vi "SetAngleCruz.vi"(0 "Time Manager Output":dbl, 1 "ta > tf/2?":bool, 2 "Angular Velocity":dbl, 3 "Time Acceleration":dbl, 4 "Time Cruise":dbl) -> (5 "Current Angle":dbl)   [LabVIEW 2015]
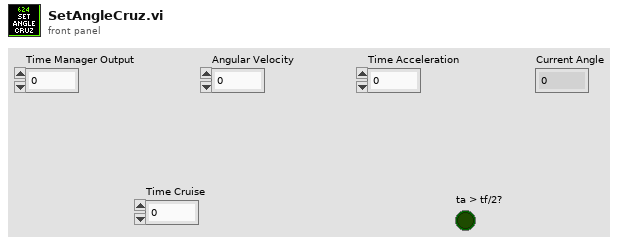
[diagram p1: front panel]
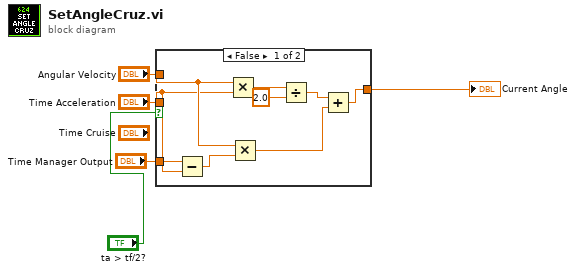
[diagram p0: block diagram]
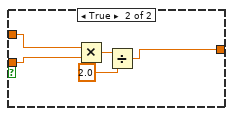
[diagram p2: hidden frame]
diagram:
  n1 = case shown="False" "ta > tf/2?" {
    tunnel: "Time Manager Output" -> [w11 _]
    tunnel: "Angular Velocity" -> [w9 w19]
    tunnel: [w7 w15] -> w3
    tunnel: "Time Acceleration" -> [w6 w18]
    frame False {
      n2 = Subtract(x=w11, y=w6) -> (x-y=w10:dbl)
      n3 = Multiply(x=w9, y=w6) -> (x*y=w14:dbl)
      n4 = Multiply(x=w9, y=w10) -> (x*y=w8:dbl)
      n5 = Divide(x=w14, y=2.0) -> (x/y=w12:dbl)
      n6 = Add(x=w12, y=w8) -> (x+y=w7:dbl)
    }
    frame True {
      n7 = Multiply(x=w19, y=w18) -> (x*y=w17:dbl)
      n8 = Divide(x=w17, y=2.0) -> (x/y=w15:dbl)
    }
  }
  "Current Angle" <- w3
